vi "Countdown.vi"(8 "error in":errorcluster, 10 "Refresh Timeout (ms)":i32=10, 11 "Countdown Time (ms)":dbl=5000.0 format="%#_13g") -> (0 "error out":errorcluster)   [LabVIEW 2018]
doc: "(<B>Filename</B>: Actor Framework.lvlib:Actor.lvclass:Actor Core.vi)\n\nReceives messages to the actor, reacts to them, and initiates any error handling that may shut the actor down.\n\nDescendant classes may override this VI to append parallel tasks for the actor to complete while it handles messages. Overrides use the Call Parent Method node."
panel:
  out "Countdown Message":string
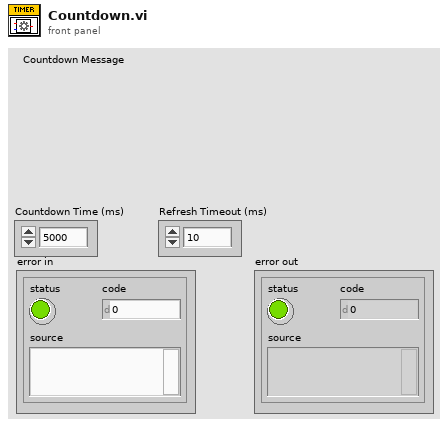
[diagram p1: front panel]
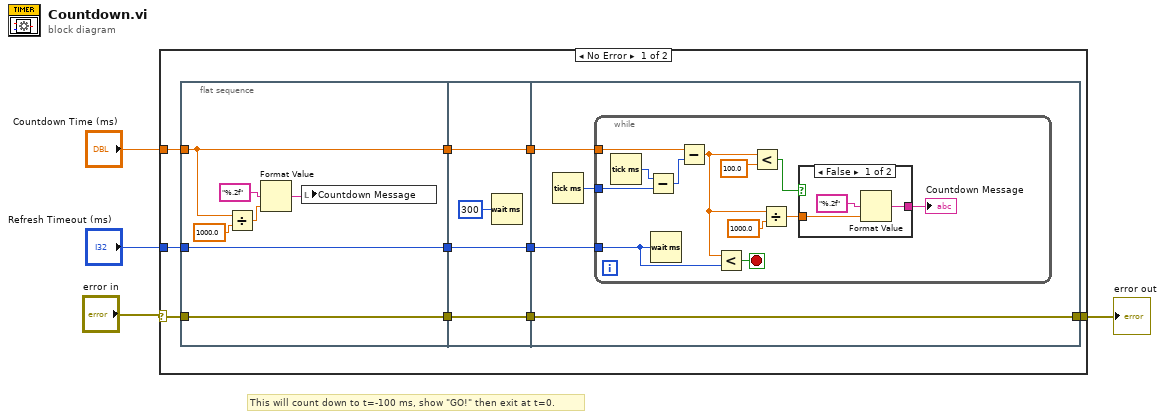
[diagram p0: block diagram]
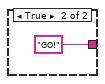
[diagram p2: hidden frame]
diagram:
  # "This will count down to t=-100 ms, show \"GO!\" then exit at t=0."
  n1 = case shown="No Error" "error in" {
    selector: "error in" -> [w12 w46]
    tunnel: "Countdown Time (ms)" -> [w14 _]
    tunnel: "Refresh Timeout (ms)" -> [w13 _]
    tunnel: [w11 w46] -> w1
    frame No Error {
      n2 = flat-sequence {
        tunnel: w13 -> [w21]
        tunnel: w14 -> [w15]
        tunnel: [w15] -> w10
        tunnel: [w21] -> w8
        tunnel: [w18] -> w6
        tunnel: w12 -> [w18]
        tunnel: w10 -> [w25]
        tunnel: [w25] -> w9
        tunnel: w8 -> [w24]
        tunnel: [w24] -> w7
        tunnel: w6 -> [w23]
        tunnel: [w23] -> w5
        tunnel: w9 -> [w28]
        tunnel: w7 -> [w27]
        tunnel: w5 -> [w26]
        tunnel: [w26] -> w11
        frame #0 {
          n3 = Divide(x=w15, y=1000.0) -> (x/y=w16:dbl)
          n4 = Format Value(format string="%.2f", value (0)=w16) -> (output string=w20:string)  [unwired: 1 in]
          n5 = local write "Countdown Message"(w20) -> ()
        }
        frame #1 {
          n6 = Wait (ms)(milliseconds to wait=u32 300) -> ()  [unwired: 1 out]
        }
        frame #2 {
          n7 = Tick Count (ms)() -> (millisecond timer value=w29:u32)
          n8 = while {
            tunnel: w29 -> [w40]
            tunnel: w28 -> [w39]
            tunnel: w27 -> [w34]
            stop <- w35 stop-if-true
            n9 = Tick Count (ms)() -> (millisecond timer value=w41:u32)
            n10 = Subtract(x=w41, y=w40) -> (x-y=w33:u32)
            n11 = Wait (ms)(milliseconds to wait=w34) -> ()  [unwired: 1 out]
            n12 = Subtract(x=w39, y=w33) -> (x-y=w30:dbl)
            n13 = Less?(x=w30, y=w34) -> (x < y?=w35:bool)
            n14 = Less?(x=w30, y=100.0) -> (x < y?=w36:bool)
            n15 = Divide(x=w30, y=1000.0) -> (x/y=w31:dbl)
            n16 = case shown="False" w36 {
              tunnel: [w43 "GO!" ("Countdown Message")] -> w38
              tunnel: w31 -> [w42 _]
              frame False {
                n17 = Format Value(format string="%.2f", value (0)=w42) -> (output string=w43:string)  [unwired: 1 in]
              }
              frame True {
              }
            }
            "Countdown Message" <- w38
          }
        }
      }
    }
    frame Error {
    }
  }
  "error out" <- w1
